vi "Hardware-System-ADC-Host.vi"() -> ()   [LabVIEW 2016]
uses:
  <vilib>/Powertrain Controls/Device Drivers/DCM/Rev0/RT/System State.ctl
  <vilib>/Powertrain Controls/Device Drivers/DCM/Rev0/RT/System ADC.ctl
  <vilib>/Powertrain Controls/Device Drivers/DCM/Rev0/RT/Internal Fault.ctl
  <vilib>/Powertrain Controls/Device Drivers/DCM/Rev0/RT/DCM - RT.lvclass
panel:
  in  "_Tabs":T1(tab)
  in  "ADC_FaultThreshLo":T2 {"Fan [V]" format="%#_3p"; "Primary B1B2 [V]" format="%#_3p"; "Primary B3B4 [V]" format="%#_3p"; "Primary A3A4 [V]" format="%#_3p"; "Primary A1A2 [V]" format="%#_3p"; "MPRD [V]" format="%#_3p"; "Ext HV B [V]" format="%#_3p"; "Ext HV A [V]" format="%#_3p"; "Pump Zener B [V]" format="%#_3p"; "Pump Zener A [V]" format="%#_3p"; "DI Zener B [V]" format="%#_3p"; "DI Zener A [V]" format="%#_3p"; "Key [V]" format="%#_3p"; "DRVP [V]" format="%#_3p"; "Battery [V]" format="%#_3p"; "FET Driver [V]" format="%#_3p"; "Secondary B1B2 [V]" format="%#_3p"; "Secondary B3B4 [V]" format="%#_3p"; "Secondary A3A4 [V]" format="%#_3p"; "Secondary A1A2 [V]" format="%#_3p"; "Primary Range [V]" format="%#_3p"; "Temp Boost B [C]" format="%#_3p"; "Temp Primary A [C]" format="%#_3p"; "Temp Secondary A [C]" format="%#_3p"; "Temp Fan Intake [C]" format="%#_3p"; "Temp CPU [C]" format="%#_3p"; "Temp DI Zener B [C]" format="%#_3p"; "Temp DI B [C]" format="%#_3p"; "Temp DI Zener A [C]" format="%#_3p"; "Temp DI A [C]" format="%#_3p"; "Temp HH 7-12 [C]" format="%#_3p"; "Temp HH 1-6 [C]" format="%#_3p"; "AI 12 [V]" format="%#_3p"; "AI 11 [V]" format="%#_3p"; "AI 10 [V]" format="%#_3p"; "AI 9 [V]" format="%#_3p"; "AI 8 [V]" format="%#_3p"; "AI 7 [V]" format="%#_3p"; "AI 6 [V]" format="%#_3p"; "AI 5 [V]" format="%#_3p"; "AI 4 [V]" format="%#_3p"; "AI 3 [V]" format="%#_3p"; "AI 2 [V]" format="%#_3p"; "AI 1 [V]" format="%#_3p"}
  out "_SystemADC":T2 {"Fan [V]" format="%#_3p"; "Primary B1B2 [V]" format="%#_3p"; "Primary B3B4 [V]" format="%#_3p"; "Primary A3A4 [V]" format="%#_3p"; "Primary A1A2 [V]" format="%#_3p"; "MPRD [V]" format="%#_3p"; "Ext HV B [V]" format="%#_3p"; "Ext HV A [V]" format="%#_3p"; "Pump Zener B [V]" format="%#_3p"; "Pump Zener A [V]" format="%#_3p"; "DI Zener B [V]" format="%#_3p"; "DI Zener A [V]" format="%#_3p"; "Key [V]" format="%#_3p"; "DRVP [V]" format="%#_3p"; "Battery [V]" format="%#_3p"; "FET Driver [V]" format="%#_3p"; "Secondary B1B2 [V]" format="%#_3p"; "Secondary B3B4 [V]" format="%#_3p"; "Secondary A3A4 [V]" format="%#_3p"; "Secondary A1A2 [V]" format="%#_3p"; "Primary Range [V]" format="%#_3p"; "Temp Boost B [C]" format="%#_3p"; "Temp Primary A [C]" format="%#_3p"; "Temp Secondary A [C]" format="%#_3p"; "Temp Fan Intake [C]" format="%#_3p"; "Temp CPU [C]" format="%#_3p"; "Temp DI Zener B [C]" format="%#_3p"; "Temp DI B [C]" format="%#_3p"; "Temp DI Zener A [C]" format="%#_3p"; "Temp DI A [C]" format="%#_3p"; "Temp HH 7-12 [C]" format="%#_3p"; "Temp HH 1-6 [C]" format="%#_3p"; "AI 12 [V]" format="%#_3p"; "AI 11 [V]" format="%#_3p"; "AI 10 [V]" format="%#_3p"; "AI 9 [V]" format="%#_3p"; "AI 8 [V]" format="%#_3p"; "AI 7 [V]" format="%#_3p"; "AI 6 [V]" format="%#_3p"; "AI 5 [V]" format="%#_3p"; "AI 4 [V]" format="%#_3p"; "AI 3 [V]" format="%#_3p"; "AI 2 [V]" format="%#_3p"; "AI 1 [V]" format="%#_3p"}
  in  "ADC_FaultThreshHi":T2 {"Fan [V]" format="%#_3p"; "Primary B1B2 [V]" format="%#_3p"; "Primary B3B4 [V]" format="%#_3p"; "Primary A3A4 [V]" format="%#_3p"; "Primary A1A2 [V]" format="%#_3p"; "MPRD [V]" format="%#_3p"; "Ext HV B [V]" format="%#_3p"; "Ext HV A [V]" format="%#_3p"; "Pump Zener B [V]" format="%#_3p"; "Pump Zener A [V]" format="%#_3p"; "DI Zener B [V]" format="%#_3p"; "DI Zener A [V]" format="%#_3p"; "Key [V]" format="%#_3p"; "DRVP [V]" format="%#_3p"; "Battery [V]" format="%#_3p"; "FET Driver [V]" format="%#_3p"; "Secondary B1B2 [V]" format="%#_3p"; "Secondary B3B4 [V]" format="%#_3p"; "Secondary A3A4 [V]" format="%#_3p"; "Secondary A1A2 [V]" format="%#_3p"; "Primary Range [V]" format="%#_3p"; "Temp Boost B [C]" format="%#_3p"; "Temp Primary A [C]" format="%#_3p"; "Temp Secondary A [C]" format="%#_3p"; "Temp Fan Intake [C]" format="%#_3p"; "Temp CPU [C]" format="%#_3p"; "Temp DI Zener B [C]" format="%#_3p"; "Temp DI B [C]" format="%#_3p"; "Temp DI Zener A [C]" format="%#_3p"; "Temp DI A [C]" format="%#_3p"; "Temp HH 7-12 [C]" format="%#_3p"; "Temp HH 1-6 [C]" format="%#_3p"; "AI 12 [V]" format="%#_3p"; "AI 11 [V]" format="%#_3p"; "AI 10 [V]" format="%#_3p"; "AI 9 [V]" format="%#_3p"; "AI 8 [V]" format="%#_3p"; "AI 7 [V]" format="%#_3p"; "AI 6 [V]" format="%#_3p"; "AI 5 [V]" format="%#_3p"; "AI 4 [V]" format="%#_3p"; "AI 3 [V]" format="%#_3p"; "AI 2 [V]" format="%#_3p"; "AI 1 [V]" format="%#_3p"}
  out "State":T3 {"System ADC"."Fan [V]" format="%#_3p"; "System ADC"."Primary B1B2 [V]" format="%#_3p"; "System ADC"."Primary B3B4 [V]" format="%#_3p"; "System ADC"."Primary A3A4 [V]" format="%#_3p"; "System ADC"."Primary A1A2 [V]" format="%#_3p"; "System ADC"."MPRD [V]" format="%#_3p"; "System ADC"."Ext HV B [V]" format="%#_3p"; "System ADC"."Ext HV A [V]" format="%#_3p"; "System ADC"."Pump Zener B [V]" format="%#_3p"; "System ADC"."Pump Zener A [V]" format="%#_3p"; "System ADC"."DI Zener B [V]" format="%#_3p"; "System ADC"."DI Zener A [V]" format="%#_3p"; "System ADC"."Key [V]" format="%#_3p"; "System ADC"."DRVP [V]" format="%#_3p"; "System ADC"."Battery [V]" format="%#_3p"; "System ADC"."FET Driver [V]" format="%#_3p"; "System ADC"."Secondary B1B2 [V]" format="%#_3p"; "System ADC"."Secondary B3B4 [V]" format="%#_3p"; "System ADC"."Secondary A3A4 [V]" format="%#_3p"; "System ADC"."Secondary A1A2 [V]" format="%#_3p"; "System ADC"."Primary Range [V]" format="%#_3p"; "System ADC"."Temp Boost B [C]" format="%#_3p"; "System ADC"."Temp Primary A [C]" format="%#_3p"; "System ADC"."Temp Secondary A [C]" format="%#_3p"; "System ADC"."Temp Fan Intake [C]" format="%#_3p"; "System ADC"."Temp CPU [C]" format="%#_3p"; "System ADC"."Temp DI Zener B [C]" format="%#_3p"; "System ADC"."Temp DI B [C]" format="%#_3p"; "System ADC"."Temp DI Zener A [C]" format="%#_3p"; "System ADC"."Temp DI A [C]" format="%#_3p"; "System ADC"."Temp HH 7-12 [C]" format="%#_3p"; "System ADC"."Temp HH 1-6 [C]" format="%#_3p"; "System ADC"."AI 12 [V]" format="%#_3p"; "System ADC"."AI 11 [V]" format="%#_3p"; "System ADC"."AI 10 [V]" format="%#_3p"; "System ADC"."AI 9 [V]" format="%#_3p"; "System ADC"."AI 8 [V]" format="%#_3p"; "System ADC"."AI 7 [V]" format="%#_3p"; "System ADC"."AI 6 [V]" format="%#_3p"; "System ADC"."AI 5 [V]" format="%#_3p"; "System ADC"."AI 4 [V]" format="%#_3p"; "System ADC"."AI 3 [V]" format="%#_3p"; "System ADC"."AI 2 [V]" format="%#_3p"; "System ADC"."AI 1 [V]" format="%#_3p"}
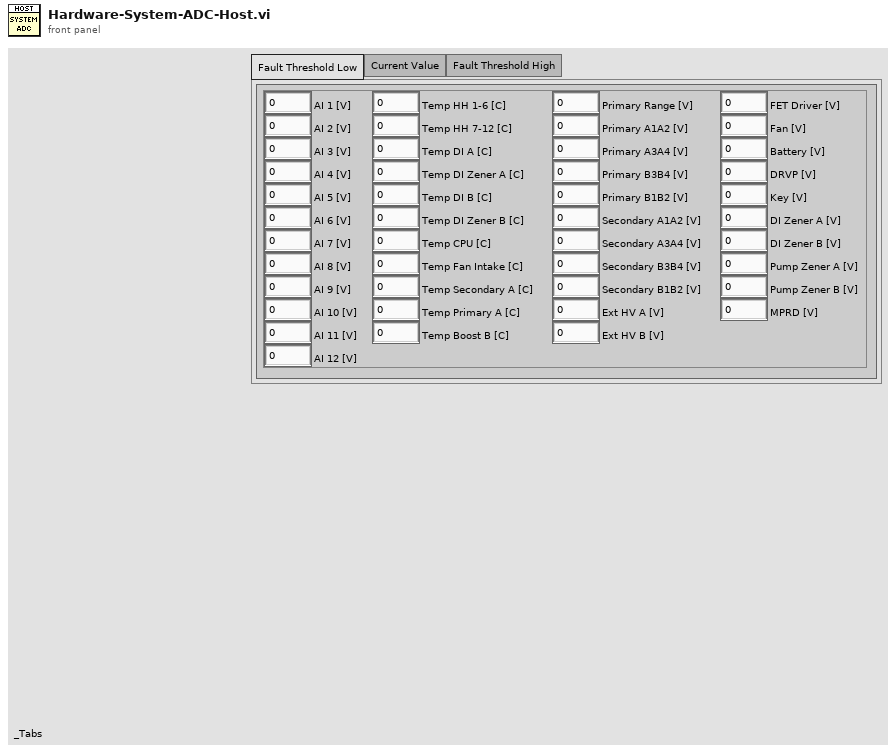
[diagram p1: front panel]
types:
  T1 = enum32{"Fault Threshold Low", "Current Value", "Fault Threshold High"}
  T2 = typedef "DCM - RT.lvclass/System ADC.ctl" = cluster{"AI 1 [V]":sgl, "AI 2 [V]":sgl, "AI 3 [V]":sgl, "AI 4 [V]":sgl, "AI 5 [V]":sgl, "AI 6 [V]":sgl, "AI 7 [V]":sgl, "AI 8 [V]":sgl, "AI 9 [V]":sgl, "AI 10 [V]":sgl, "AI 11 [V]":sgl, "AI 12 [V]":sgl, "Temp HH 1-6 [C]":sgl, "Temp HH 7-12 [C]":sgl, "Temp DI A [C]":sgl, "Temp DI Zener A [C]":sgl, "Temp DI B [C]":sgl, "Temp DI Zener B [C]":sgl, "Temp CPU [C]":sgl, "Temp Fan Intake [C]":sgl, "Temp Secondary A [C]":sgl, "Temp Primary A [C]":sgl, "Temp Boost B [C]":sgl, "Primary Range [V]":sgl, "Primary A1A2 [V]":sgl, "Primary A3A4 [V]":sgl, "Primary B3B4 [V]":sgl, "Primary B1B2 [V]":sgl, "Secondary A1A2 [V]":sgl, "Secondary A3A4 [V]":sgl, "Secondary B3B4 [V]":sgl, "Secondary B1B2 [V]":sgl, "Ext HV A [V]":sgl, "Ext HV B [V]":sgl, "FET Driver [V]":sgl, "Fan [V]":sgl, "Battery [V]":sgl, "DRVP [V]":sgl, "Key [V]":sgl, "DI Zener A [V]":sgl, "DI Zener B [V]":sgl, "Pump Zener A [V]":sgl, "Pump Zener B [V]":sgl, "MPRD [V]":sgl}
  T3 = typedef "DCM - RT.lvclass/System State.ctl" = cluster{"System ADC":T2, "IO Lock":bool, "HH Mode Config Error":bool, "Fan Speed 1 [RPM]":sgl, "Fan Speed 2 [RPM]":sgl, "Firmware Major Rev":u16, "Firmware Minor Rev":u16, "Internal Fault":T4, "Fault Value":dbl}
  T4 = typedef "DCM - RT.lvclass/Internal Fault.ctl" = enum32{"None", "Temp HH 1-6", "Temp HH 7-12", "Temp DI A", "Temp DI Zener A", "Temp DI B", "Temp DI Zener B", "Temp Intake", "Temp Primary A", "Temp Secondary A", "Temp Boost B", "Temp CPU", "Low Battery", "Inrush Protection", "A Run Enable", "B Run Enable", "Fan Speed"}
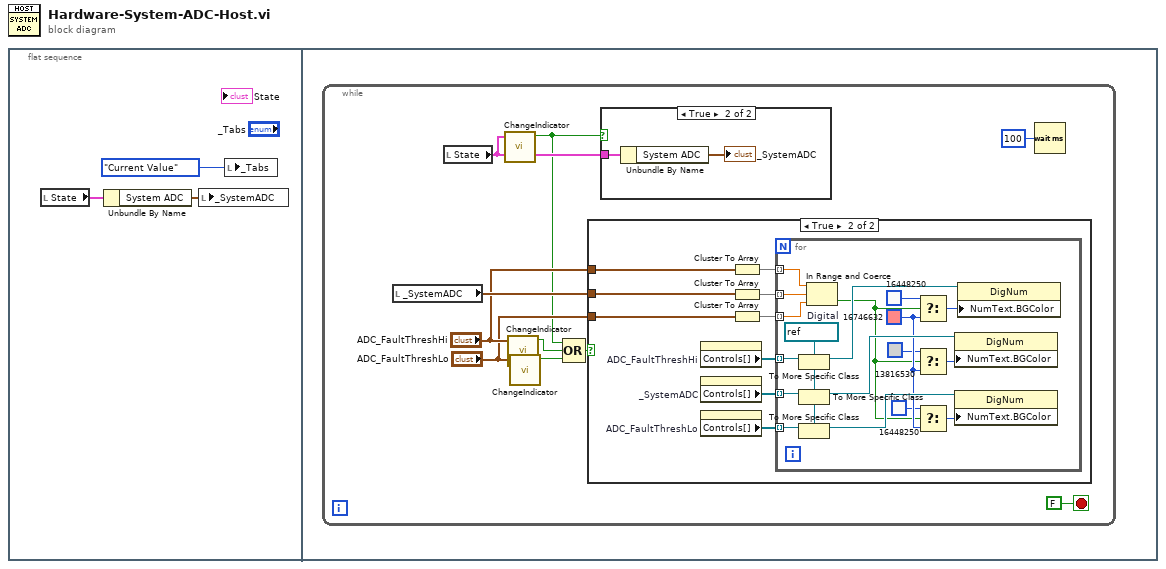
[diagram p0: block diagram]
diagram:
  n1 = flat-sequence {
    frame #0 {
      n2 = local read "State"() -> (w2:T3)
      n3 = Unbundle By Name(w2) -> ("System ADC"=w3:T2)
      n4 = local write "_SystemADC"(w3) -> ()
      n5 = local write "_Tabs"(T1."Current Value" ("Tab Control")) -> ()
    }
    frame #1 {
      n6 = while {
        stop <- FALSE stop-if-true
        n7 = local read "_SystemADC"() -> (w10:T2)
        n8 = local read "State"() -> (w11:T3)
        n9 = call "ChangeIndicator.vi"("Input"=w11) -> ("Change"=w4:bool)  [unwired: 9 in]
        n10 = call "ChangeIndicator.vi"("Input"="ADC_FaultThreshHi") -> ("Change"=w6:bool)  [unwired: 9 in]
        n11 = call "ChangeIndicator.vi"("Input"="ADC_FaultThreshLo") -> ("Change"=w5:bool)  [unwired: 9 in]
        n12 = Compound Arithmetic op=OR(w4, w6, w5) -> (w7:bool)
        n13 = case shown="True" w7 {
          tunnel: w10 -> [_ w22]
          tunnel: "ADC_FaultThreshHi" -> [_ w15]
          tunnel: "ADC_FaultThreshLo" -> [_ w14]
          frame False {
          }
          frame True {
            n14 = property on="ADC_FaultThreshHi" class="Clust (strict)"() -> ("Controls[]"=w17:refnum<vi>[])  [unwired: 2 in, 2 out]
            n15 = property on="_SystemADC" class="Clust (strict)"() -> ("Controls[]"=w16:refnum<vi>[])  [unwired: 2 in, 2 out]
            n16 = property on="ADC_FaultThreshLo" class="Clust (strict)"() -> ("Controls[]"=w18:refnum<vi>[])  [unwired: 2 in, 2 out]
            n17 = Cluster To Array(cluster=w15) -> (array=w19:sgl[])
            n18 = Cluster To Array(cluster=w22) -> (array=w21:sgl[])
            n19 = Cluster To Array(cluster=w14) -> (array=w20:sgl[])
            n20 = for {
              tunnel: w21 -> [w38] mode=indexing
              tunnel: w20 -> [w36] mode=indexing
              tunnel: w19 -> [w37] mode=indexing
              tunnel: w18 -> [w40] mode=indexing
              tunnel: w17 -> [w39] mode=indexing
              tunnel: w16 -> [w35] mode=indexing
              w27 = u32 16746632
              w31 = refnum<vi> refnum  # Digital
              n21 = To More Specific Class(target class=w31, reference=w39) -> (specific class reference=w34:refnum<vi>)  [unwired: 1 in, 1 out]
              n22 = To More Specific Class(target class=w31, reference=w35) -> (specific class reference=w33:refnum<vi>)  [unwired: 1 in, 1 out]
              n23 = To More Specific Class(target class=w31, reference=w40) -> (specific class reference=w32:refnum<vi>)  [unwired: 1 in, 1 out]
              n24 = In Range and Coerce(upper limit=w37, x=w38, lower limit=w36) -> (In Range?=w26:bool)  [unwired: 1 out]
              n25 = Select(t=u32 16448250, s=w26, f=w27) -> (s? t:f=w30:u32)
              n26 = Select(t=u32 13816530, s=w26, f=w27) -> (s? t:f=w28:u32)
              n27 = Select(t=u32 16448250, s=w26, f=w27) -> (s? t:f=w29:u32)
              n28 = property class="DigNum"(reference=w33, "NumText.BGColor"=w28) -> ()  [unwired: 1 in, 2 out]
              n29 = property class="DigNum"(reference=w32, "NumText.BGColor"=w29) -> ()  [unwired: 1 in, 2 out]
              n30 = property class="DigNum"(reference=w34, "NumText.BGColor"=w30) -> ()  [unwired: 1 in, 2 out]
            }
          }
        }
        n31 = case shown="True" w4 {
          tunnel: w11 -> [_ w42]
          frame False {
          }
          frame True {
            n32 = Unbundle By Name(w42) -> ("System ADC"=→"_SystemADC":T2)
          }
        }
        n33 = Wait (ms)(milliseconds to wait=u32 100) -> ()  [unwired: 1 out]
      }
    }
  }
